vi "buffer.vi"(8 "dimension size":i32=10, 11 "input":dbl) -> (3 "delayed input":dbl)   [LabVIEW 2018]
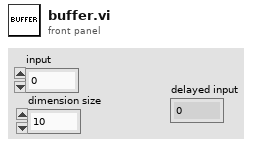
[diagram p1: front panel]
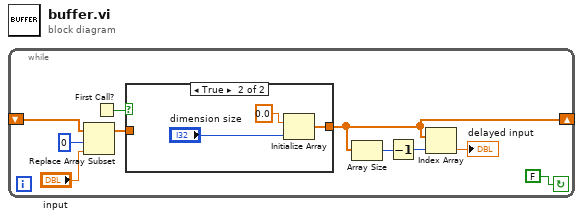
[diagram p0: block diagram]
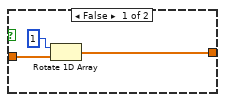
[diagram p2: hidden frame]
diagram:
  n1 = while {
    shift-right: [w3] -> _
    shift-left: _ -> [w7]
    stop <- FALSE continue-if-true
    n2 = Replace Array Subset(array=w7, new element="input", index=0) -> (w5:dbl[])
    n3 = First Call?() -> (First Call?: T/F=w9:bool)
    n4 = case shown="True" w9 {
      tunnel: [w13 w15] -> w3
      tunnel: w5 -> [w12 _]
      frame False {
        n5 = Rotate 1D Array(1:w12, 2:1 ("n")) -> (0:w13:dbl[])
      }
      frame True {
        n6 = Initialize Array(0.0 ("element"), "dimension size") -> (w15:dbl[])
      }
    }
    n7 = Array Size(array=w3) -> (size(s)=w2:i32)
    n8 = Decrement(x=w2) -> (x-1=w1:i32)
    n9 = Index Array(array=w3, index=w1) -> (element=→"delayed input":dbl)
  }
